vi "表达式节点.vi"() -> ()   [LabVIEW 2010]
panel:
  out "输出y":dbl
  in  "输入x":dbl
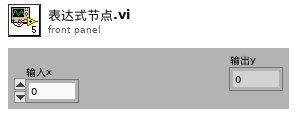
[diagram p1: front panel]
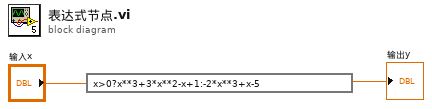
[diagram p0: block diagram]
diagram:
  n1 = expression code="x>0?x**3+3*x**2-x+1:-2*x**3+x-5"("输入x") -> (→"输出y":dbl)
